vi "XNET_HighVoltage_Read.vi"() -> ()   [LabVIEW 2022 SP3]
uses:
  <vilib>/xnet/xnet.llb/XNET Create Session (Signal Output Single-point).vi
  <vilib>/xnet/xnet.llb/XNET Write (Signal Single-point).vi
  <vilib>/xnet/xnet.llb/XNET Read (Signal Single-point).vi
panel:
  out "error out":errorcluster
  out "data":dbl[](array[numeric]) format="%.2f"
  in  "error in (no error)":errorcluster
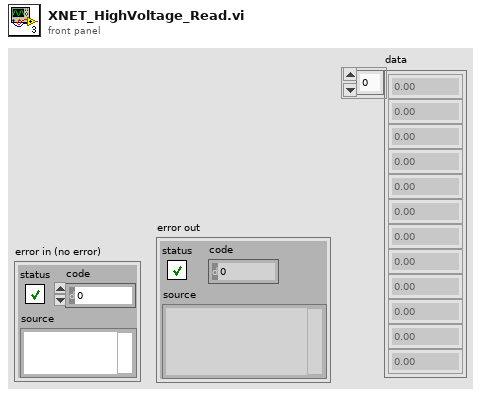
[diagram p1: front panel]
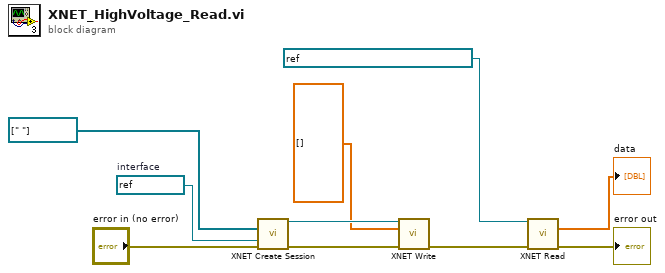
[diagram p0: block diagram]
diagram:
  w9 = refnum<k21> "CAN1"  # interface
  n1 = call-poly <vilib>:"XNET Create Session.vi"("signal list"=refnum<k21>[] [" "], "interface"=w9, "error in (no error)"="error in (no error)") -> ("session out"=w10:refnum<k21>, "error out"=w8:errorcluster)  [unwired: 11 in]
  n2 = call-poly <vilib>:"XNET Write.vi"("session in"=w10, "data"=dbl[] [], "error in (no error)"=w8) -> ("error out"=w7:errorcluster)  [unwired: 11 in, 1 out]
  n3 = call-poly <vilib>:"XNET Read.vi"("session in"=refnum<k21> "FTS2_HV_CANSessionPD500BZ", "error in (no error)"=w7) -> ("data"=→"data":dbl[], "error out"=→"error out":errorcluster)  [unwired: 11 in, 1 out]
